vi "IV_Forward.vi"(3 "error in (no error)":errorcluster, 4 "Input cluster":T1={"Vmin"=0.001, "Vmax"=0.001, "Step"=0.001, "milliseconds to wait"=10, "limit current [mA]"=0.001, "ms to ramp down"=10, "Stop"=FALSE} {"ms to ramp down" format="%#_13g"; "Vmax" format="%#_13g"}, 5 "Upper Measurement Range":u16(ring)=2 items=["20mA", "2mA", "200uA", "20uA", "2uA", "200nA", "20nA", "2nA"], 6 "VISA Keithley resource in":refnum<visa-resource-name>) -> (0 "error out":errorcluster, 1 "IV cluster":cluster{dbl[], dbl[]}, 2 "VISA Keithley resource out":refnum<visa-resource-name>)   [LabVIEW 2022 SP3]
uses:
  IV_cluster_in.ctl
  <instrlib>/Keithley 648X Series/Keithley 648X Series.lvlib
panel:
  out "XY Graph 2":cluster{dbl[], dbl[]}(graph)
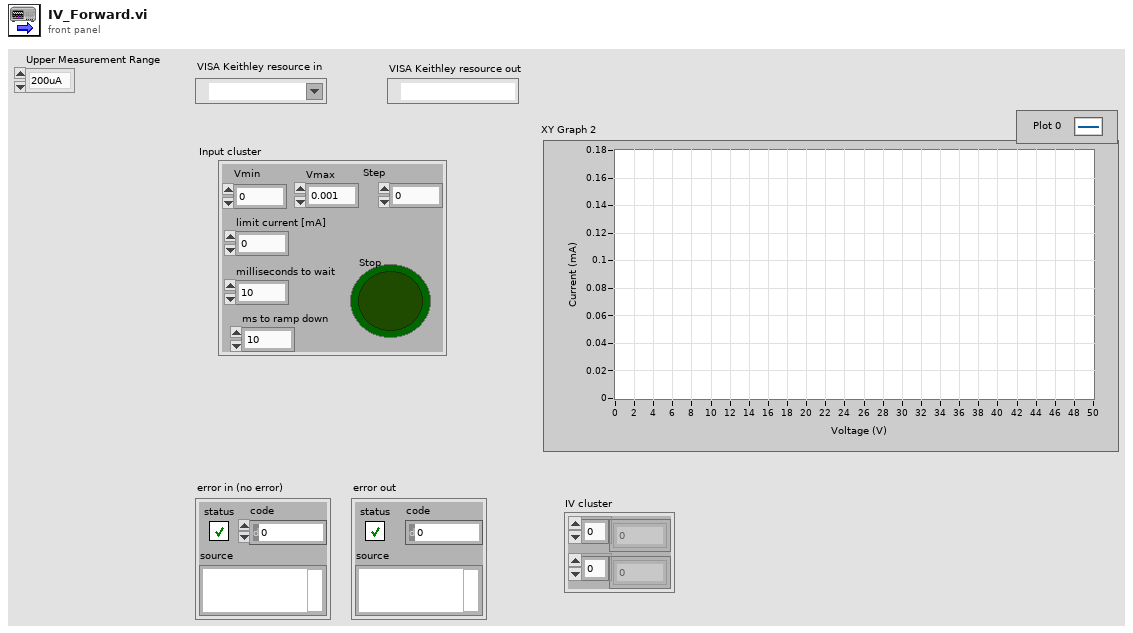
[diagram p1: front panel]
types:
  T1 = typedef "IV_cluster_in.ctl" = cluster{"Vmin":dbl, "Vmax":dbl, "Step":dbl, "milliseconds to wait":u32, "limit current [mA]":dbl, "ms to ramp down":u32, "Stop":bool}
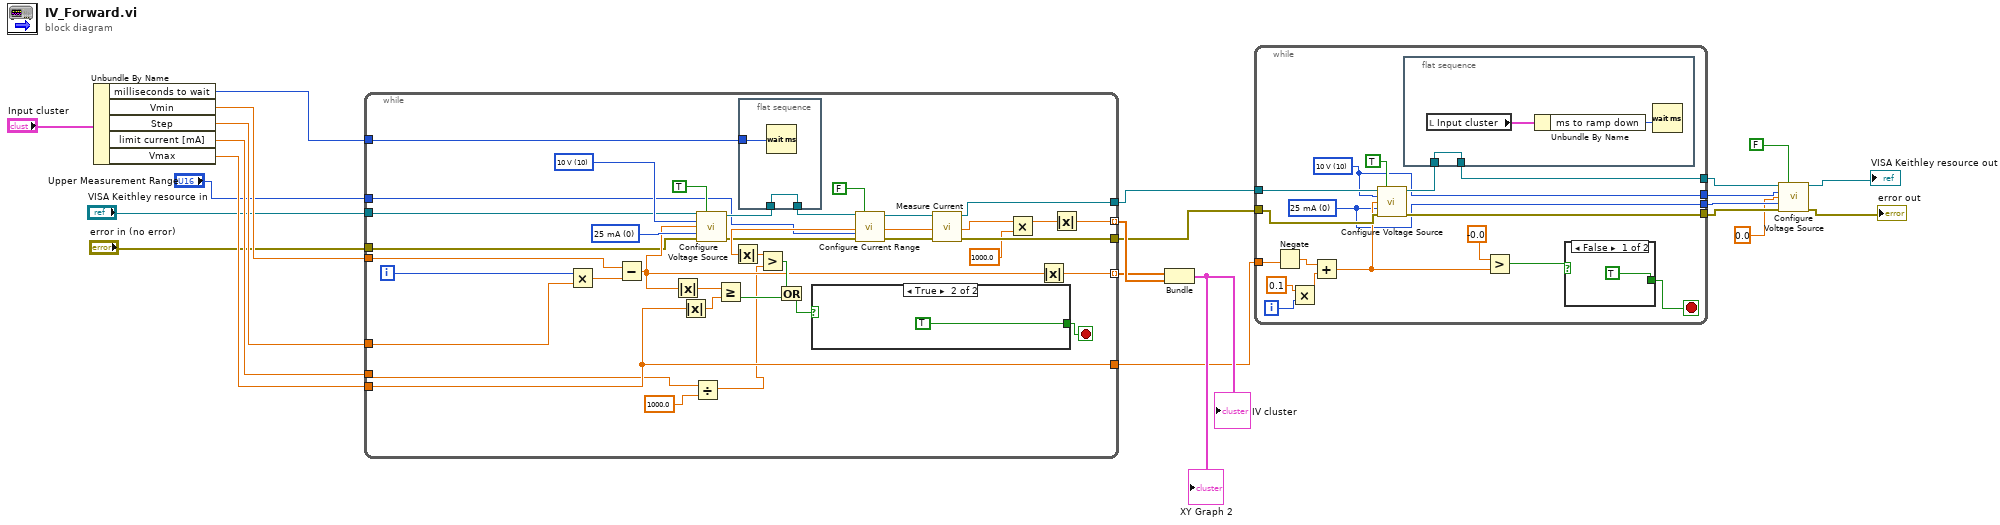
[diagram p0: block diagram]
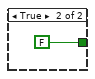
[diagram p2: hidden frame]
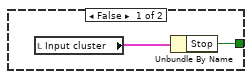
[diagram p3: hidden frame]
diagram:
  n1 = Unbundle By Name("Input cluster") -> ("milliseconds to wait"=w12:u32, "Vmin"=w16:dbl, "Step"=w15:dbl, "limit current [mA]"=w14:dbl, "Vmax"=w13:dbl)
  n2 = while {
    tunnel: [w41] -> w23 mode=indexing
    tunnel: [w59] -> w20
    tunnel: [w58] -> w19
    tunnel: w16 -> [w57]
    tunnel: [w42] -> w22 mode=indexing
    tunnel: [w35] -> w18
    tunnel: w15 -> [w36]
    tunnel: w14 -> [w34]
    tunnel: w13 -> [w35]
    tunnel: w12 -> [w40]
    tunnel: "VISA Keithley resource in" -> [w38]
    tunnel: "error in (no error)" -> [w37]
    tunnel: "Upper Measurement Range" -> [w25]
    i -> [w50]
    stop <- w39 stop-if-true
    w55 = u16 10 items=["10 V"=10, "50 V"=50, "500 V"=500] ("Voltage Source Range (10 V)")
    w56 = u16 0 items=["25 mA", "2.5 mA", "250 uA", "25 uA"] ("Current Limit (25 mA)")
    n3 = Multiply(x=w50, y=w36) -> (x*y=w51:dbl)
    n4 = Subtract(x=w57, y=w51) -> (x-y=w43:dbl)
    n5 = Absolute Value(x=w43) -> (abs(x)=w45:dbl)
    n6 = Absolute Value(x=w35) -> (abs(x)=w44:dbl)
    n7 = Divide(x=w34, y=1000.0) -> (x/y=w33:dbl)
    n8 = call <instrlib>:"Configure Voltage Source.vi"("VISA resource name"=w38, "Enable Voltage Source (F: Disable)"=TRUE, "Voltage Source Range (10 V)"=w55, "Voltage Level (0 V)"=w43, "Current Limit (25 mA)"=w56, "error in (no error)"=w37) -> ("VISA resource name out"=w49:refnum<visa-resource-name>, "error out"=w26:errorcluster)  [unwired: 8 in]
    n9 = Greater Or Equal?(x=w45, y=w44) -> (x >= y?=w46:bool)
    n10 = flat-sequence {
      tunnel: w49 -> [w61]
      tunnel: [w61] -> w27
      tunnel: w40 -> [w60]
      frame #0 {
        n11 = Wait (ms)(milliseconds to wait=w60) -> ()  [unwired: 1 out]
      }
    }
    n12 = call <instrlib>:"Configure Current Range.vi"("VISA resource name"=w27, "Autorange (T: Enable)"=FALSE, "Upper Measurement Range (200uA)"=w25, "error in (no error)"=w26) -> ("VISA resource name out"=w29:refnum<visa-resource-name>, "error out"=w28:errorcluster)  [unwired: 10 in]
    n13 = call <instrlib>:"Measure Current.vi"("VISA resource name"=w29, "error in (no error)"=w28) -> ("VISA resource name out"=w59:refnum<visa-resource-name>, "Measurement"=w30:dbl, "error out"=w58:errorcluster)  [unwired: 11 in]
    n14 = Absolute Value(x=w30) -> (abs(x)=w31:dbl)
    n15 = Greater?(x=w31, y=w33) -> (0:w54:bool)
    n16 = Or(x=w54, y=w46) -> (x .or. y?=w53:bool)
    n17 = case shown="True" w53 {
      tunnel: [w63 TRUE] -> w39
      frame False {
        n18 = local read "Input cluster"() -> (w62:T1)
        n19 = Unbundle By Name(w62) -> ("Stop"=w63:bool)
      }
      frame True {
      }
    }
    n20 = Multiply(x=w30, y=1000.0) -> (x*y=w48:dbl)
    n21 = Absolute Value(x=w43) -> (abs(x)=w42:dbl)
    n22 = Absolute Value(x=w48) -> (abs(x)=w41:dbl)
  }
  n23 = Bundle(w22, w23) -> (→"XY Graph 2" →"IV cluster":cluster{dbl[], dbl[]})  [unwired: 1 in]
  n24 = while {
    tunnel: w20 -> [w80]
    tunnel: [w78] -> w9
    tunnel: w19 -> [w77]
    tunnel: [w76] -> w8
    tunnel: w18 -> [w66]
    tunnel: [w68] -> w5
    tunnel: [w67] -> w4
    i -> [w70]
    stop <- w72 stop-if-true
    w68 = u16 10 items=["10 V"=10, "50 V"=50, "500 V"=500] ("Voltage Source Range (10 V)")
    w67 = u16 0 items=["25 mA", "2.5 mA", "250 uA", "25 uA"] ("Current Limit (25 mA)")
    n25 = Negate(x=w66) -> (-x=w65:dbl)
    n26 = Multiply(x=0.1, y=w70) -> (x*y=w69:dbl)
    n27 = Add(x=w65, y=w69) -> (x+y=w74:dbl)
    n28 = call <instrlib>:"Configure Voltage Source.vi"("VISA resource name"=w80, "Enable Voltage Source (F: Disable)"=TRUE, "Voltage Source Range (10 V)"=w68, "Voltage Level (0 V)"=w74, "Current Limit (25 mA)"=w67, "error in (no error)"=w77) -> ("VISA resource name out"=w79:refnum<visa-resource-name>, "error out"=w76:errorcluster)  [unwired: 8 in]
    n29 = flat-sequence {
      tunnel: w79 -> [w84]
      tunnel: [w84] -> w78
      frame #0 {
        n30 = local read "Input cluster"() -> (w82:T1)
        n31 = Unbundle By Name(w82) -> ("ms to ramp down"=w83:u32)
        n32 = Wait (ms)(milliseconds to wait=w83) -> ()  [unwired: 1 out]
      }
    }
    n33 = Greater?(x=-0.0 ("Step"), y=w74) -> (0:w73:bool)
    n34 = case shown="False" w73 {
      tunnel: [TRUE FALSE] -> w72
      frame False {
      }
      frame True {
      }
    }
  }
  n35 = call <instrlib>:"Configure Voltage Source.vi"("VISA resource name"=w9, "Enable Voltage Source (F: Disable)"=FALSE, "Voltage Source Range (10 V)"=w5, "Voltage Level (0 V)"=0.0, "Current Limit (25 mA)"=w4, "error in (no error)"=w8) -> ("VISA resource name out"=→"VISA Keithley resource out":refnum<visa-resource-name>, "error out"=→"error out":errorcluster)  [unwired: 8 in]
